vi "convert-sce-cmd-list.vi"(11 "sce-cmd-list":cluster{"字符串":string, "数组 2":string[]}[](array[cluster])) -> (3 "场景-cmd-list":T2(array[cluster]))   [LabVIEW 2019]
panel:
  out "场景 2":T1
  out "场景":T1
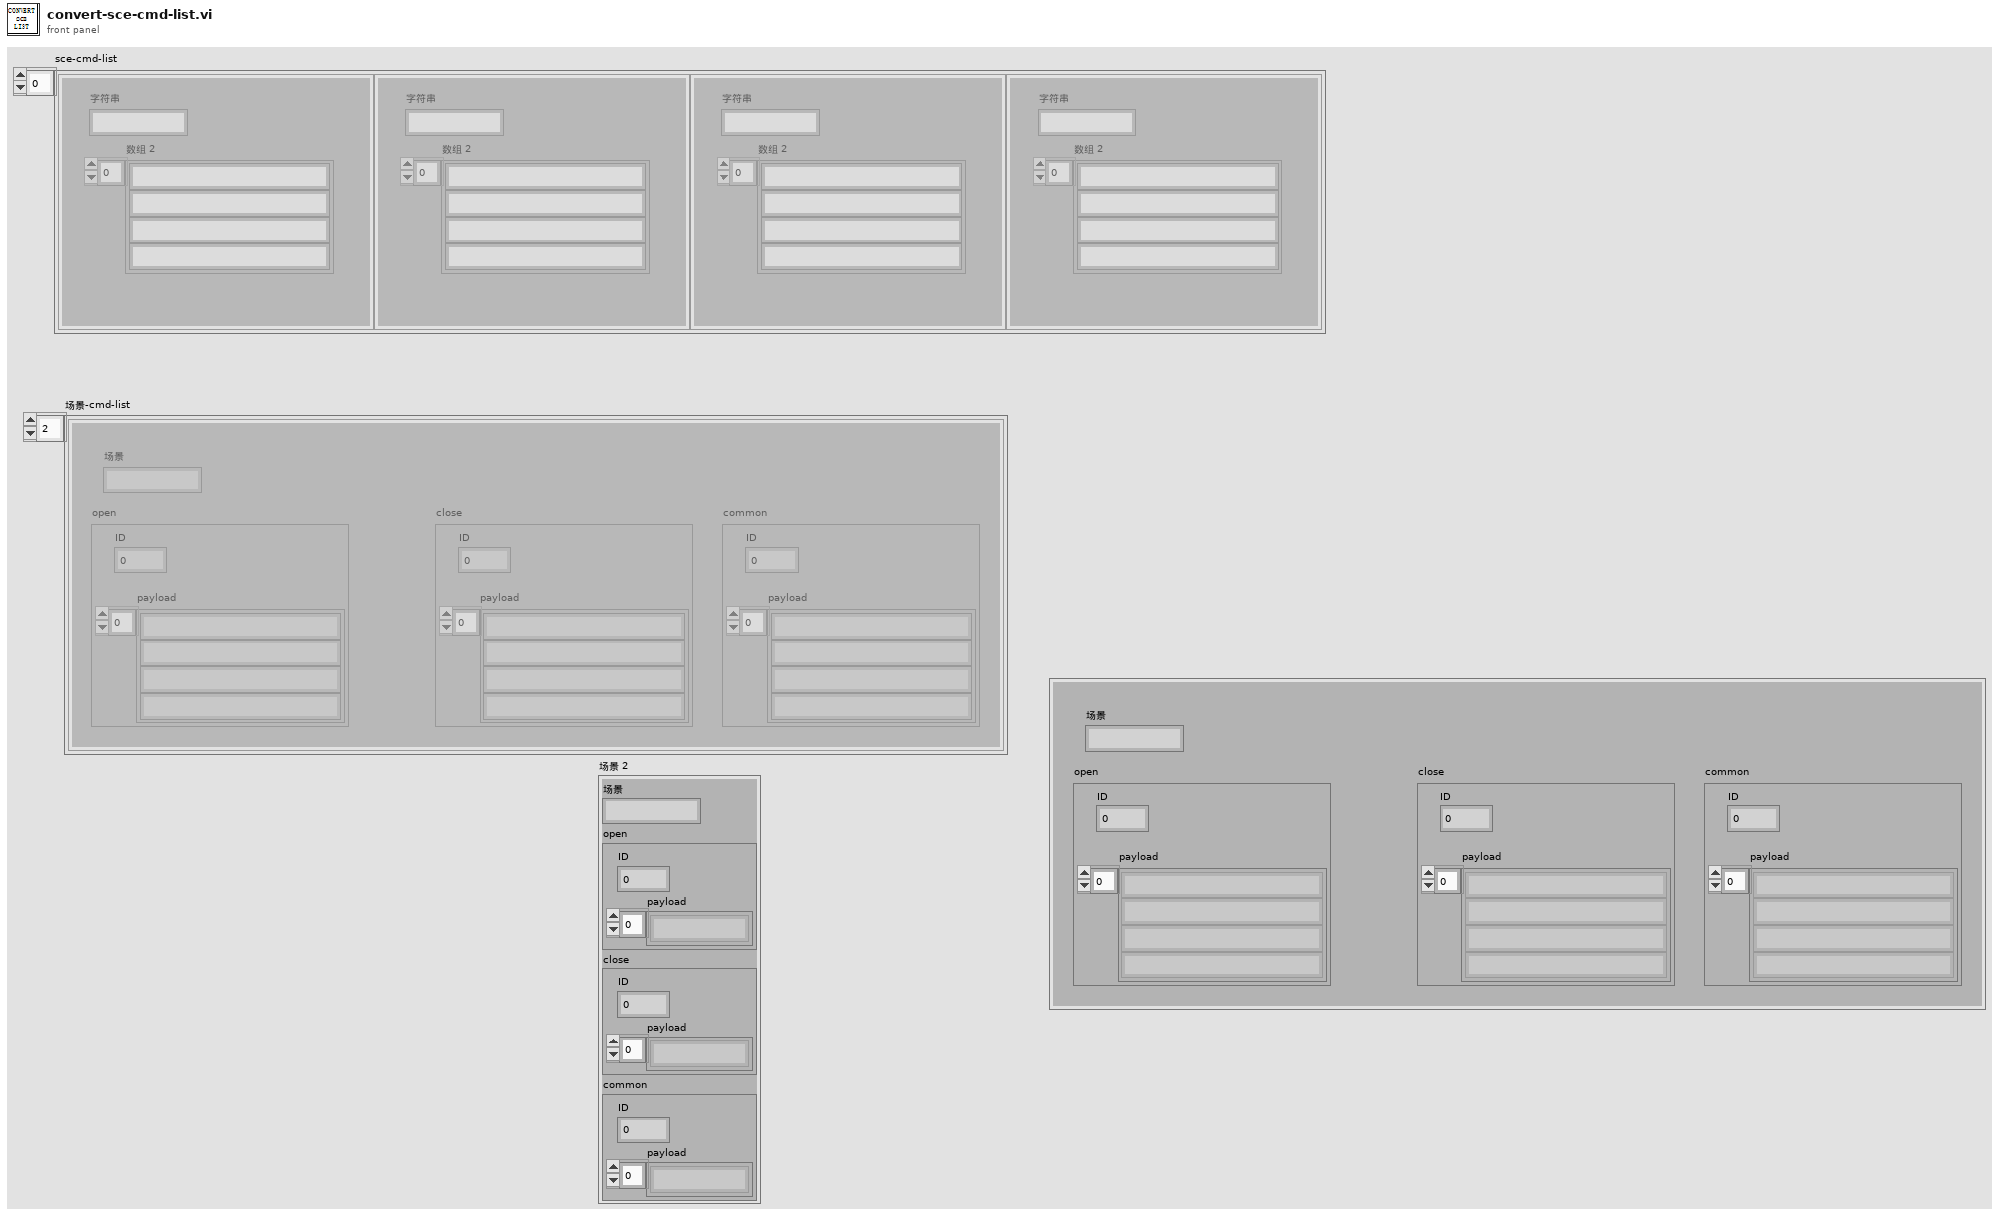
[diagram p1: front panel]
types:
  T1 = cluster{"场景":string, "open":cluster{"ID":dbl, "payload":string[]}, "close":cluster{"ID":dbl, "payload":string[]}, "common":cluster{"ID":dbl, "payload":string[]}}
  T2 = cluster{"场景":string, "open":cluster{"ID":dbl, "payload":string[]}, "close":cluster{"ID":dbl, "payload":string[]}, "common":cluster{"ID":dbl, "payload":string[]}}[]
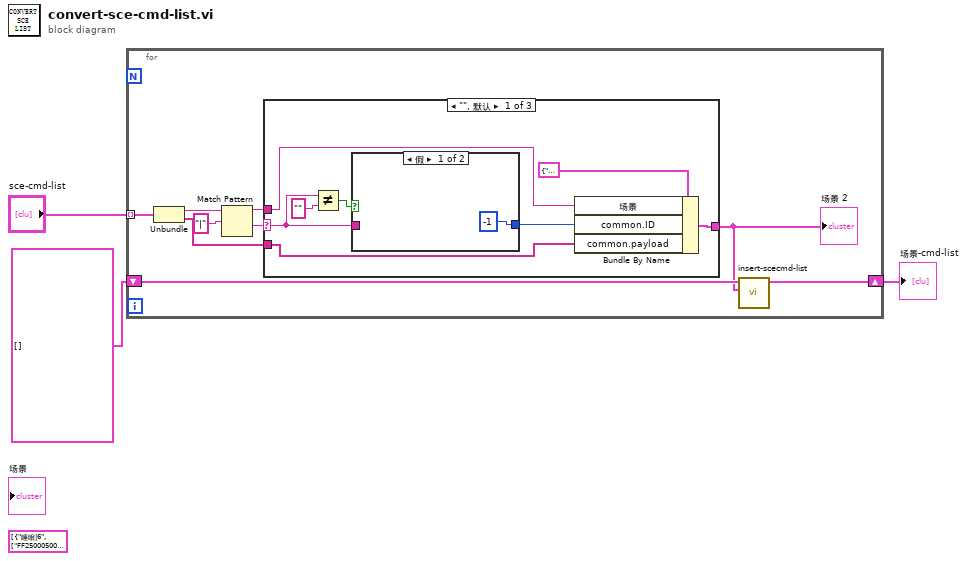
[diagram p0: block diagram]
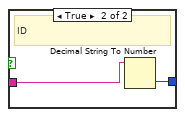
[diagram p2: hidden frame]
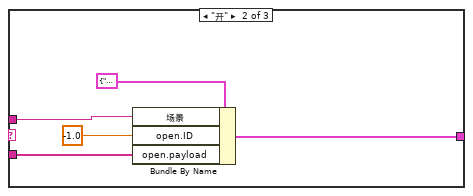
[diagram p3: hidden frame]
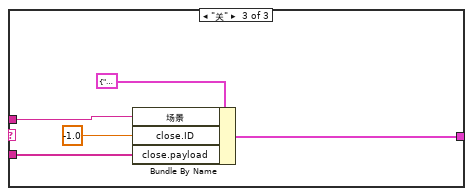
[diagram p4: hidden frame]
diagram:
  (unwired) cluster{"字符串":string, "数组 2":string[]}[] [{"字符串"="睡眠|6", "数组 2"=["FF2500050003030103010301"]}, {"字符串"="起床|开", "数组 2"=["FF25000700010301"]}, {"字符串"="起床|关", "数组 2"=["FF250006000203010100"]}] ("sce-cmd-list")
  n1 = for {
    tunnel: "sce-cmd-list" -> [w12] mode=indexing
    shift-right: [w4] -> w1
    shift-left: T2 [] ("场景-cmd-list") -> [w6]
    n2 = Unbundle(w12) -> ("字符串"=w11:string, "数组 2"=w8:string[])
    n3 = Match Pattern(string=w11, regular expression="|" ("正则表达式")) -> (before substring=w7:string, after substring=w9:string)  [unwired: 1 in, 2 out]
    n4 = case shown="\"\", 默认" w9 {
      selector: w9 -> [w18 _ _]
      tunnel: w8 -> [w15 w25 w30]
      tunnel: w7 -> [w16 w26 w31]
      tunnel: [w13 w24 w29] -> w5
      frame "", Default {
        n5 = Not Equal?(x=w18, y="") -> (x != y?=w19:bool)
        n6 = case shown="假" w19 {
          tunnel: w18 -> [_ w23]
          tunnel: [-1 w22] -> w14
          frame False {
          }
          frame True {
            # "ID"
            n7 = Decimal String To Number(string=w23) -> (number=w22:i32)  [unwired: 2 in, 1 out]
          }
        }
        n8 = Bundle By Name(cluster=T1 {"场景"="", "open"={"ID"=0.0, "payload"=[]}, "close"={"ID"=0.0, "payload"=[]}, "common"={"ID"=0.0, "payload"=[]}} ("场景"), "场景"=w16, "common.ID"=w14, "common.payload"=w15) -> (w13:T1)
      }
      frame "开" {
        n9 = Bundle By Name(cluster=T1 {"场景"="", "open"={"ID"=0.0, "payload"=[]}, "close"={"ID"=0.0, "payload"=[]}, "common"={"ID"=0.0, "payload"=[]}} ("场景"), "场景"=w26, "open.ID"=-1.0 ("common.ID"), "open.payload"=w25) -> (w24:T1)
      }
      frame "关" {
        n10 = Bundle By Name(cluster=T1 {"场景"="", "open"={"ID"=0.0, "payload"=[]}, "close"={"ID"=0.0, "payload"=[]}, "common"={"ID"=0.0, "payload"=[]}} ("场景"), "场景"=w31, "close.ID"=-1.0 ("common.ID"), "close.payload"=w30) -> (w29:T1)
      }
    }
    "场景 2" <- w5
    n11 = call "insert-scecmd-list.vi"("场景"=w5, "场景-cmd-list"=w6) -> ("场景-cmd-list out"=w4:T2)  [unwired: 9 in]
  }
  "场景-cmd-list" <- w1
